vi "AlGaInPAs_prep_run_cont_v09.vi"(2 "Debug Mode":bool, 3 "Elapsed Time(s)":dbl, 4 "State":enum16{"Edit", "Start", "Run", "End", "Idle"}(ring), 5 "Argument List In":string[](array[string])) -> (0 "Status Out":string, 1 "Argument List Out":string[](array[string]))   [LabVIEW 2011]
panel:
  out "prep_done":bool
  out "run started":bool
  out "first":bool=TRUE
  out "total time":dbl
  out "is OK?":bool
  out "AsH3?":bool
  out "PH3?":bool
  out "In?":bool
  out "Ga?":bool
  out "Al?":bool
  in  "Prep As":bool caption="Pre-run"
  in  "Prep P":bool caption="Pre-run"
  in  "Prep In":bool caption="Pre-run"
  in  "Prep Ga":bool caption="Pre-run"
  in  "prep_time":dbl caption="pre-run time (s)"
  in  "Prep Al":bool caption="Pre-run"
  in  "Run As":bool caption="Run"
  in  "AsH3 Flow":dbl caption="AsH3 Flow (0-10 sccm)" format="%.2f"
  in  "P Flow":dbl caption="P Flow (0-100 sccm)" format="%.2f"
  in  "Run P":bool caption="Run"
  in  "In Flow":dbl caption="In Flow (0-100 sscm)" format="%.2f"
  in  "Run In":bool caption="Run"
  in  "Run Ga":bool caption="Run"
  in  "Ga Flow":dbl caption="Ga Flow (0-10 sscm)" format="%.2f"
  in  "Run Al":bool caption="Run"
  in  "Al Flow":dbl caption="Al Flow (0-100 sscm)" format="%.2f"
  in  "Cancel":bool
  in  "OK":bool
  out "tTotal(s) 2":dbl
  # "Add pre-run time to run time in editor."
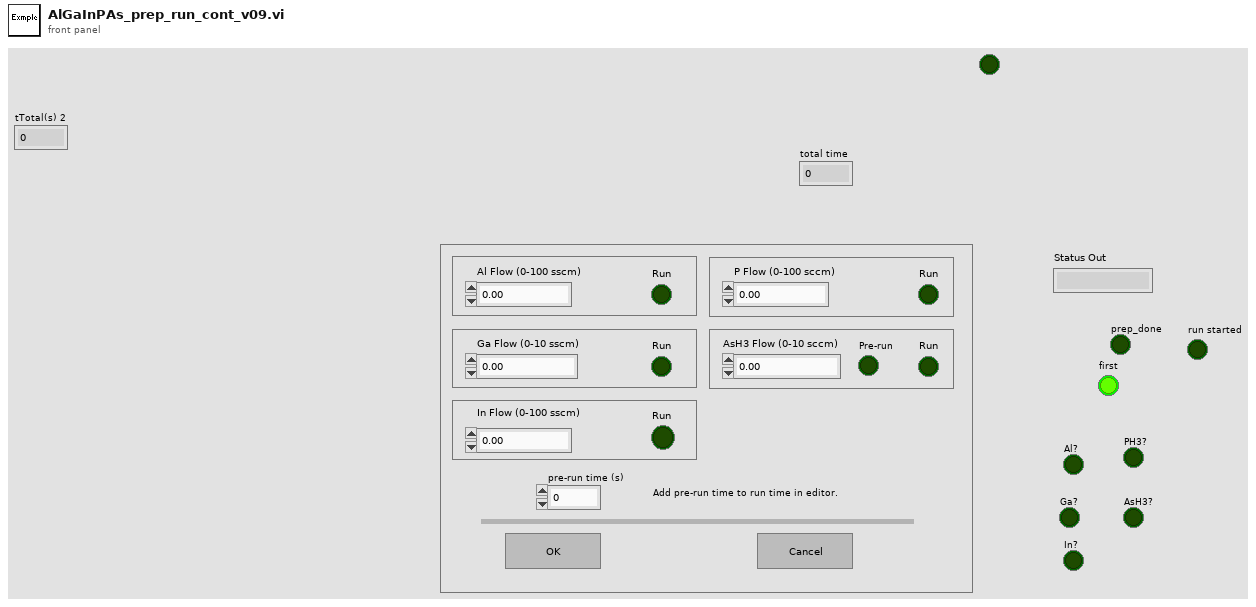
[diagram p1: front panel]
types:
  T1 = enum16{"Discrete", "Continuous", "Instantaneous", "Finite"}
  T2 = enum32{"Invalid", "Default", "Floating", "Floating/Auto-Hide", "Modal"}
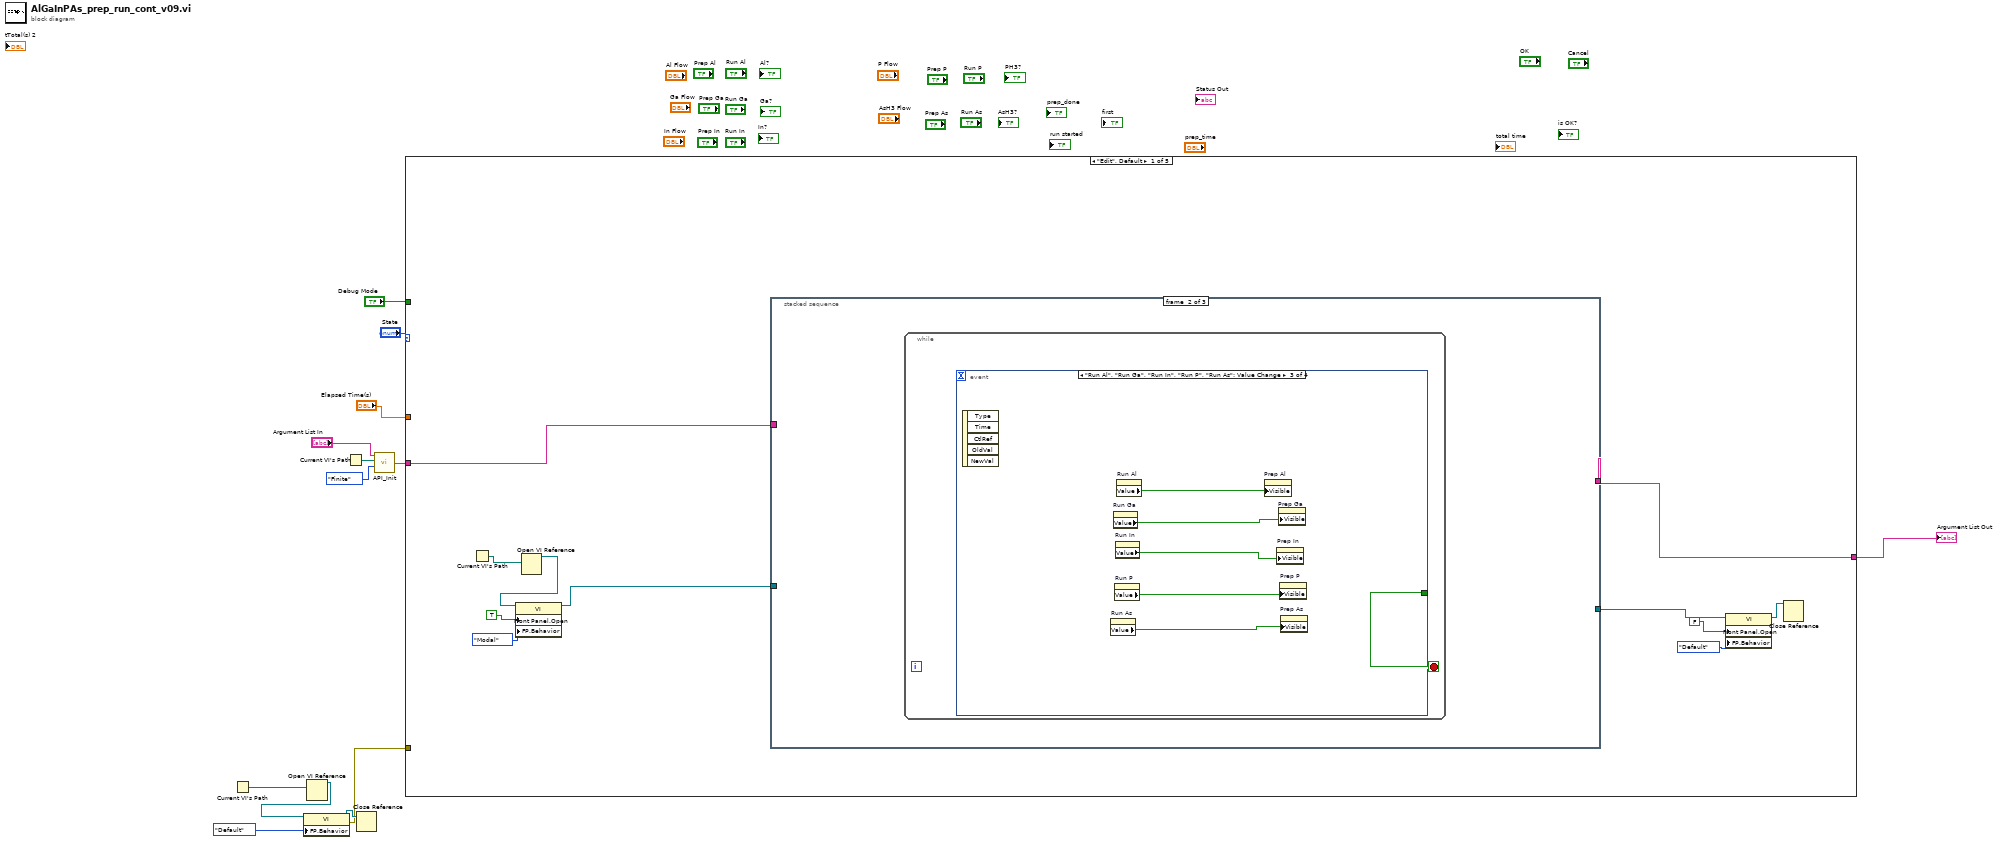
[diagram p0: block diagram]
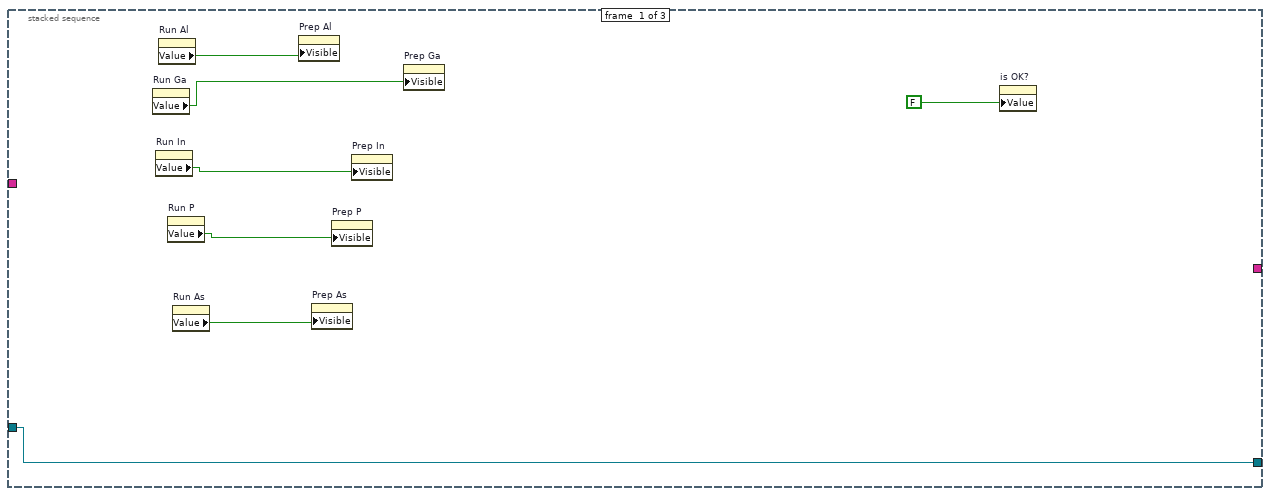
[diagram p2: hidden frame]
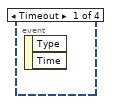
[diagram p3: hidden frame]
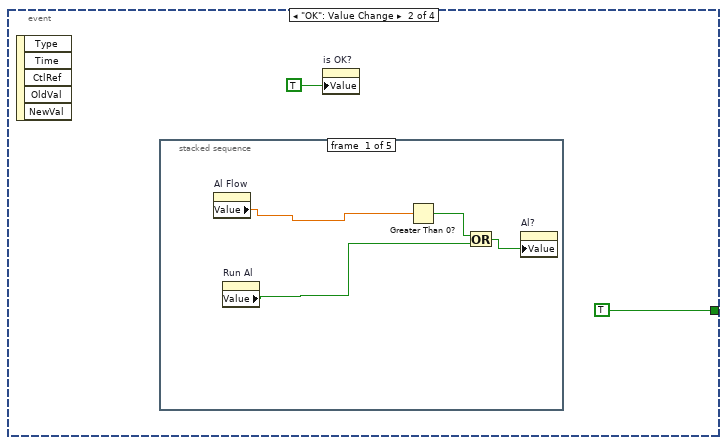
[diagram p4: hidden frame]
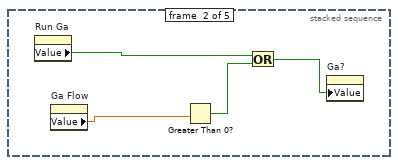
[diagram p5: hidden frame]
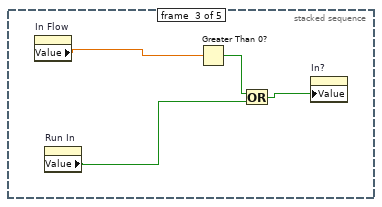
[diagram p6: hidden frame]
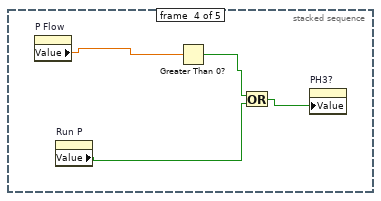
[diagram p7: hidden frame]
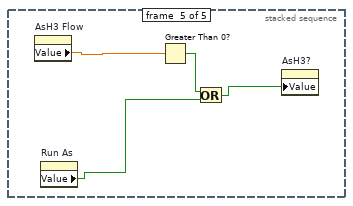
[diagram p8: hidden frame]
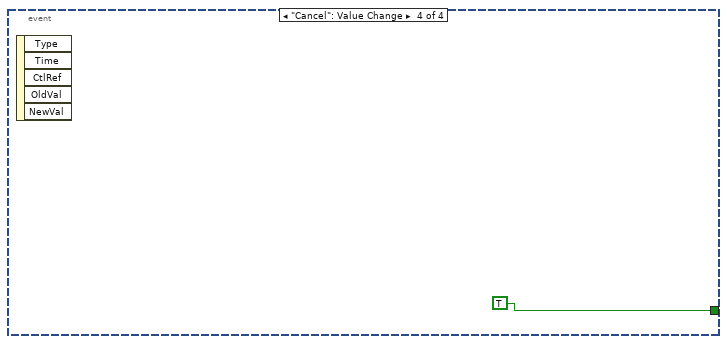
[diagram p9: hidden frame]
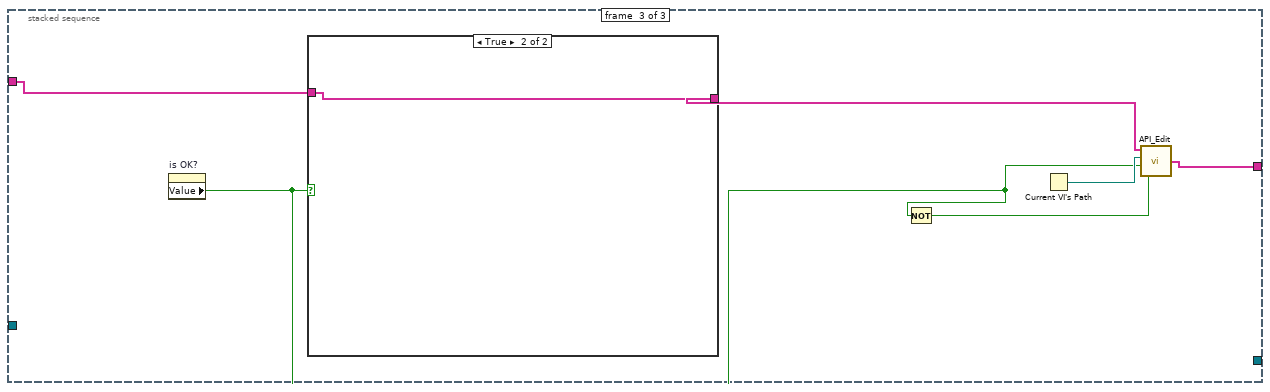
[diagram p10: hidden frame]
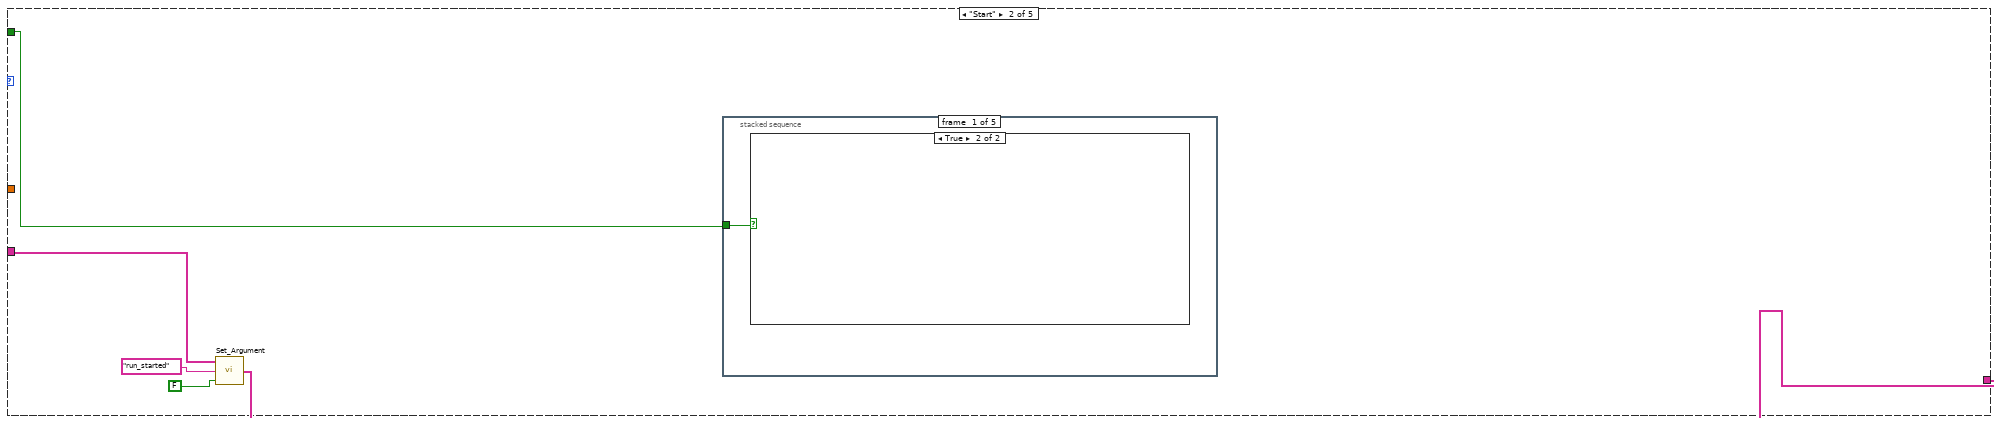
[diagram p12: hidden frame]
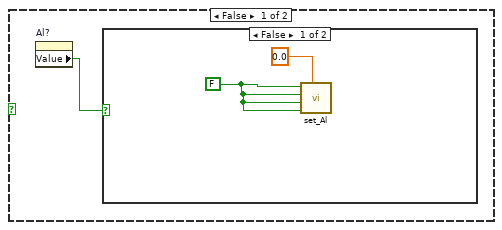
[diagram p13: hidden frame]
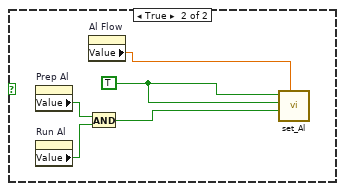
[diagram p14: hidden frame]
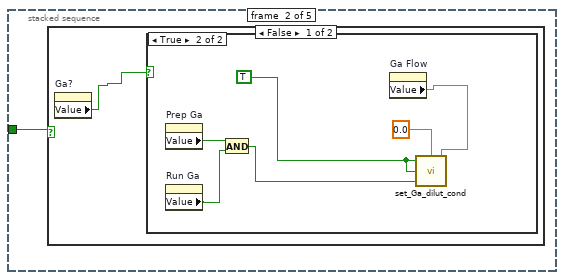
[diagram p15: hidden frame]
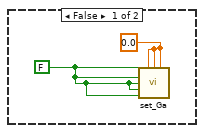
[diagram p16: hidden frame]
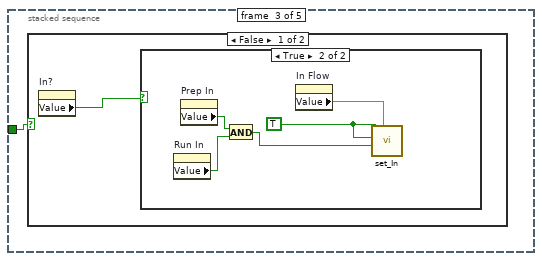
[diagram p18: hidden frame]
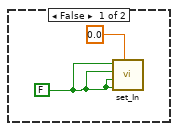
[diagram p19: hidden frame]
diagram:
  n1 = Current VI's Path() -> (path=w9:path)
  n2 = Open VI Reference(vi path=w9) -> (vi reference=w8:refnum<vi>)  [unwired: 1 in, 5 out]
  n3 = property class="VI"(reference=w8, "FP.Behavior"=T2."Default" ("Front Panel Window:Behavior")) -> (reference out=w6:refnum<vi>, error out=w5:errorcluster)  [unwired: 1 in]
  n4 = Current VI's Path() -> (path=w4:path)
  n5 = Close Reference(reference=w6) -> ()  [unwired: 1 in, 1 out]
  n6 = call "API_Init.vi"("API Mode"=T1."Finite", "VI Path"=w4, "Argument List In"="Argument List In") -> ("Argument List Out"=w1:string[])  [unwired: 1 in]
  n7 = case shown="\"Edit\", Default" "State" {
    tunnel: "Debug Mode" -> [_ w69 w121 _ _]
    tunnel: "Elapsed Time(s)" -> [_ _ w123 _ _]
    tunnel: w1 -> [w15 w71 w120 w236 w237]
    tunnel: [w14 w70 w122 w236 w237] -> w10
    tunnel: w5 -> [_ _ _ _ _]
    frame "Edit", Default {
      n8 = Current VI's Path() -> (path=w20:path)
      n9 = Open VI Reference(vi path=w20) -> (vi reference=w19:refnum<vi>)  [unwired: 1 in, 5 out]
      n10 = property class="VI"(reference=w19, "Front Panel.Open"=TRUE ("Front Panel Window:Open"), "FP.Behavior"=T2."Modal" ("Front Panel Window:Behavior")) -> (reference out=w18:refnum<vi>)  [unwired: 1 in, 1 out]
      n11 = stacked-sequence {
        tunnel: w15 -> [_ _ w64]
        tunnel: w18 -> [w31 _ _]
        tunnel: [w31 _ _] -> w22
        tunnel: [_ _ w62] -> w14
        frame #0 {
          n12 = property on="Run Ga" class="Bool (strict)"() -> ("Value"=w28:bool)  [unwired: 2 in, 2 out]
          n13 = property on="Run In" class="Bool (strict)"() -> ("Value"=w27:bool)  [unwired: 2 in, 2 out]
          n14 = property on="Run Al" class="Bool (strict)"() -> ("Value"=w29:bool)  [unwired: 2 in, 2 out]
          n15 = property on="Run P" class="Bool (strict)"() -> ("Value"=w26:bool)  [unwired: 2 in, 2 out]
          n16 = property on="Run As" class="Bool (strict)"() -> ("Value"=w25:bool)  [unwired: 2 in, 2 out]
          n17 = property on="Prep Al" class="Bool (strict)"("Visible"=w29) -> ()  [unwired: 2 in, 2 out]
          n18 = property on="Prep As" class="Bool (strict)"("Visible"=w25) -> ()  [unwired: 2 in, 2 out]
          n19 = property on="Prep P" class="Bool (strict)"("Visible"=w26) -> ()  [unwired: 2 in, 2 out]
          n20 = property on="Prep In" class="Bool (strict)"("Visible"=w27) -> ()  [unwired: 2 in, 2 out]
          n21 = property on="Prep Ga" class="Bool (strict)"("Visible"=w28) -> ()  [unwired: 2 in, 2 out]
          n22 = property on="is OK?" class="Bool (strict)"("Value"=FALSE ("is OK?")) -> ()  [unwired: 2 in, 2 out]
        }
        frame #1 {
          n23 = while {
            stop <- w32 stop-if-true
            n24 = event shown="[2] \"Run Al\", \"Run Ga\", \"Run In\", \"Run P\", \"Run As\": Value Change" {
              selector: _ -> [_ _ _ _]
              dyn-events: _ -> [_ _ _ _]
              timeout: _ -> [_ _ _ _]
              tunnel: [_ TRUE _ TRUE] -> w32
              event Timeout {
                n25 = event-data() -> ()  [unwired: 1 in, 2 out]
              }
              event "OK": Value Change {
                n26 = event-data() -> ()  [unwired: 1 in, 5 out]
                n27 = stacked-sequence {
                  frame #0 {
                    n28 = property on="Al Flow" class="DigNum (strict)"() -> ("Value"=w37:dbl)  [unwired: 2 in, 2 out]
                    n29 = property on="Run Al" class="Bool (strict)"() -> ("Value"=w36:bool)  [unwired: 2 in, 2 out]
                    n30 = Greater Than 0?(x=w37) -> (x > 0?=w38:bool)
                    n31 = Or(x=w38, y=w36) -> (x .or. y?=w35:bool)
                    n32 = property on="Al?" class="Bool (strict)"("Value"=w35) -> ()  [unwired: 2 in, 2 out]
                  }
                  frame #1 {
                    n33 = property on="Run Ga" class="Bool (strict)"() -> ("Value"=w40:bool)  [unwired: 2 in, 2 out]
                    n34 = property on="Ga Flow" class="DigNum (strict)"() -> ("Value"=w41:dbl)  [unwired: 2 in, 2 out]
                    n35 = Greater Than 0?(x=w41) -> (x > 0?=w42:bool)
                    n36 = Or(x=w40, y=w42) -> (x .or. y?=w39:bool)
                    n37 = property on="Ga?" class="Bool (strict)"("Value"=w39) -> ()  [unwired: 2 in, 2 out]
                  }
                  frame #2 {
                    n38 = property on="In Flow" class="DigNum (strict)"() -> ("Value"=w44:dbl)  [unwired: 2 in, 2 out]
                    n39 = property on="Run In" class="Bool (strict)"() -> ("Value"=w45:bool)  [unwired: 2 in, 2 out]
                    n40 = Greater Than 0?(x=w44) -> (x > 0?=w46:bool)
                    n41 = Or(x=w46, y=w45) -> (x .or. y?=w43:bool)
                    n42 = property on="In?" class="Bool (strict)"("Value"=w43) -> ()  [unwired: 2 in, 2 out]
                  }
                  frame #3 {
                    n43 = property on="P Flow" class="DigNum (strict)"() -> ("Value"=w49:dbl)  [unwired: 2 in, 2 out]
                    n44 = property on="Run P" class="Bool (strict)"() -> ("Value"=w48:bool)  [unwired: 2 in, 2 out]
                    n45 = Greater Than 0?(x=w49) -> (x > 0?=w50:bool)
                    n46 = Or(x=w50, y=w48) -> (x .or. y?=w47:bool)
                    n47 = property on="PH3?" class="Bool (strict)"("Value"=w47) -> ()  [unwired: 2 in, 2 out]
                  }
                  frame #4 {
                    n48 = property on="AsH3 Flow" class="DigNum (strict)"() -> ("Value"=w53:dbl)  [unwired: 2 in, 2 out]
                    n49 = property on="Run As" class="Bool (strict)"() -> ("Value"=w52:bool)  [unwired: 2 in, 2 out]
                    n50 = Greater Than 0?(x=w53) -> (x > 0?=w54:bool)
                    n51 = Or(x=w54, y=w52) -> (x .or. y?=w51:bool)
                    n52 = property on="AsH3?" class="Bool (strict)"("Value"=w51) -> ()  [unwired: 2 in, 2 out]
                  }
                }
                n53 = property on="is OK?" class="Bool (strict)"("Value"=TRUE ("is OK?")) -> ()  [unwired: 2 in, 2 out]
              }
              event "Run Al", "Run Ga", "Run In", "Run P", "Run As": Value Change {
                n54 = event-data() -> ()  [unwired: 1 in, 5 out]
                n55 = property on="Run As" class="Bool (strict)"() -> ("Value"=w59:bool)  [unwired: 2 in, 2 out]
                n56 = property on="Run Ga" class="Bool (strict)"() -> ("Value"=w56:bool)  [unwired: 2 in, 2 out]
                n57 = property on="Run P" class="Bool (strict)"() -> ("Value"=w58:bool)  [unwired: 2 in, 2 out]
                n58 = property on="Run In" class="Bool (strict)"() -> ("Value"=w57:bool)  [unwired: 2 in, 2 out]
                n59 = property on="Run Al" class="Bool (strict)"() -> ("Value"=w55:bool)  [unwired: 2 in, 2 out]
                n60 = property on="Prep Al" class="Bool (strict)"("Visible"=w55) -> ()  [unwired: 2 in, 2 out]
                n61 = property on="Prep In" class="Bool (strict)"("Visible"=w57) -> ()  [unwired: 2 in, 2 out]
                n62 = property on="Prep Ga" class="Bool (strict)"("Visible"=w56) -> ()  [unwired: 2 in, 2 out]
                n63 = property on="Prep P" class="Bool (strict)"("Visible"=w58) -> ()  [unwired: 2 in, 2 out]
                n64 = property on="Prep As" class="Bool (strict)"("Visible"=w59) -> ()  [unwired: 2 in, 2 out]
              }
              event "Cancel": Value Change {
                n65 = event-data() -> ()  [unwired: 1 in, 5 out]
              }
            }
          }
        }
        frame #2 {
          n66 = property on="is OK?" class="Bool (strict)"() -> ("Value"=w61:bool)  [unwired: 2 in, 2 out]
          n67 = case shown="True" w61 {
            tunnel: w64 -> [w67 w68]
            tunnel: [w67 w68] -> w63
            frame False {
            }
            frame True {
            }
          }
          n68 = Not(x=w61) -> (.not. x?=w66:bool)
          n69 = Current VI's Path() -> (path=w65:path)
          n70 = call "API_Edit.vi"("Cancel"=w66, "OK"=w61, "VI Path"=w65, "Argument List In"=w63) -> ("Argument List Out"=w62:string[])
        }
      }
      n71 = property class="VI"(reference=w22, "Front Panel.Open"=FALSE ("Front Panel Window:Open"), "FP.Behavior"=T2."Default" ("Front Panel Window:Behavior")) -> (reference out=w23:refnum<vi>)  [unwired: 1 in, 1 out]
      n72 = Close Reference(reference=w23) -> ()  [unwired: 1 in, 1 out]
    }
    frame "Start" {
      n73 = call "Set_Argument.vi"("Enable"=FALSE, "Argument"="run_started", "Argument List In"=w71) -> ("Argument List Out"=w70:string[])
      n74 = stacked-sequence {
        tunnel: w69 -> [w74 w83 w93 w102 w111]
        frame #0 {
          n75 = case shown="True" w74 {
            frame False {
              n76 = property on="Al?" class="Bool (strict)"() -> ("Value"=w75:bool)  [unwired: 2 in, 2 out]
              n77 = case shown="False" w75 {
                frame False {
                  w76 = FALSE ("Al Active")
                  n78 = call "set_Al.vi"("Aluminum Flow"=0.0, "Al Remote"=w76, "Al Run"=w76, "Al Bubbler"=w76, "Al Active"=w76) -> ()  [unwired: 5 out]
                }
                frame True {
                  w82 = TRUE ("Al Active")
                  n79 = property on="Prep Al" class="Bool (strict)"() -> ("Value"=w80:bool)  [unwired: 2 in, 2 out]
                  n80 = property on="Run Al" class="Bool (strict)"() -> ("Value"=w79:bool)  [unwired: 2 in, 2 out]
                  n81 = property on="Al Flow" class="DigNum (strict)"() -> ("Value"=w81:dbl)  [unwired: 2 in, 2 out]
                  n82 = And(x=w80, y=w79) -> (x .and. y?=w78:bool)
                  n83 = call "set_Al.vi"("Aluminum Flow"=w81, "Al Run"=w78, "Al Bubbler"=w82, "Al Active"=w82) -> ()  [unwired: 1 in, 5 out]
                }
              }
            }
            frame True {
            }
          }
        }
        frame #1 {
          n84 = case shown="False" w83 {
            frame False {
              n85 = property on="Ga?" class="Bool (strict)"() -> ("Value"=w84:bool)  [unwired: 2 in, 2 out]
              n86 = case shown="True" w84 {
                frame False {
                  w86 = FALSE ("Ga Active")
                  w85 = 0.0 ("Ga Flow 1")
                  n87 = call "set_Ga.vi"("Ga Active"=w86, "Ga Flow 3"=w85, "Ga Flow 2"=w85, "Ga Flow 1"=w85, "Ga Bubbler"=w86, "Ga H2 Dilute"=w86, "Ga Run"=w86, "Ga Remote"=w86) -> ()  [unwired: 8 out]
                }
                frame True {
                  w92 = TRUE ("Ga Active")
                  n88 = property on="Prep Ga" class="Bool (strict)"() -> ("Value"=w89:bool)  [unwired: 2 in, 2 out]
                  n89 = property on="Run Ga" class="Bool (strict)"() -> ("Value"=w88:bool)  [unwired: 2 in, 2 out]
                  n90 = And(x=w89, y=w88) -> (x .and. y?=w87:bool)
                  n91 = property on="Ga Flow" class="DigNum (strict)"() -> ("Value"=w90:dbl)  [unwired: 2 in, 2 out]
                  n92 = call "set_Ga_dilut_cond.vi"("Ga flow (0-10 sccm)"=w90, "fDilution"=0.0, "Run"=w87, "Bubbler In"=w92, "Active"=w92) -> ()
                }
              }
            }
            frame True {
            }
          }
        }
        frame #2 {
          n93 = case shown="False" w93 {
            frame False {
              n94 = property on="In?" class="Bool (strict)"() -> ("Value"=w94:bool)  [unwired: 2 in, 2 out]
              n95 = case shown="True" w94 {
                frame False {
                  w96 = FALSE ("In Remote")
                  n96 = call "set_In.vi"("Indium Flow"=0.0, "In Remote"=w96, "In Run"=w96, "In Bubbler"=w96, "In Active"=w96) -> ()  [unwired: 5 out]
                }
                frame True {
                  w101 = TRUE ("In Run")
                  n97 = property on="Run In" class="Bool (strict)"() -> ("Value"=w98:bool)  [unwired: 2 in, 2 out]
                  n98 = property on="Prep In" class="Bool (strict)"() -> ("Value"=w99:bool)  [unwired: 2 in, 2 out]
                  n99 = And(x=w99, y=w98) -> (x .and. y?=w97:bool)
                  n100 = property on="In Flow" class="DigNum (strict)"() -> ("Value"=w100:dbl)  [unwired: 2 in, 2 out]
                  n101 = call "set_In.vi"("Indium Flow"=w100, "In Run"=w97, "In Bubbler"=w101, "In Active"=w101) -> ()  [unwired: 1 in, 5 out]
                }
              }
            }
            frame True {
            }
          }
        }
        frame #3 {
          n102 = case shown="False" w102 {
            frame False {
              n103 = property on="PH3?" class="Bool (strict)"() -> ("Value"=w103:bool)  [unwired: 2 in, 2 out]
              n104 = case shown="True" w103 {
                frame False {
                  w104 = FALSE ("P_Gas Active")
                  n105 = call "set_P_gas.vi"("P_Gas Active"=w104, "P_Gas Flow"=0.0, "P_Gas In"=w104, "P_Gas H2 In"=w104, "P_Gas Run"=w104, "P_Gas Remote"=w104) -> ()  [unwired: 10 out]
                }
                frame True {
                  w110 = TRUE ("P_Gas Active")
                  n106 = property on="P Flow" class="DigNum (strict)"() -> ("Value"=w109:dbl)  [unwired: 2 in, 2 out]
                  n107 = property on="Prep P" class="Bool (strict)"() -> ("Value"=w108:bool)  [unwired: 2 in, 2 out]
                  n108 = property on="Run P" class="Bool (strict)"() -> ("Value"=w107:bool)  [unwired: 2 in, 2 out]
                  n109 = And(x=w108, y=w107) -> (x .and. y?=w106:bool)
                  n110 = call "set_P_gas.vi"("P_Gas Active"=w110, "P_Gas Flow"=w109, "P_Gas In"=w110, "P_Gas Run"=w106) -> ()  [unwired: 2 in, 10 out]
                }
              }
            }
            frame True {
            }
          }
        }
        frame #4 {
          n111 = case shown="False" w111 {
            frame False {
              n112 = property on="AsH3?" class="Bool (strict)"() -> ("Value"=w112:bool)  [unwired: 2 in, 2 out]
              n113 = case shown="True" w112 {
                frame False {
                  w113 = FALSE ("As_Gas Active")
                  n114 = call "set_As_gas.vi"("As_Gas Active"=w113, "As_Gas Flow"=0.0, "As_Gas In"=w113, "As_Gas H2"=w113, "As_Gas Run"=w113, "As_Gas Remote"=w113) -> ()  [unwired: 10 in]
                }
                frame True {
                  w119 = TRUE ("As_Gas Active")
                  n115 = property on="Prep As" class="Bool (strict)"() -> ("Value"=w116:bool)  [unwired: 2 in, 2 out]
                  n116 = property on="Run As" class="Bool (strict)"() -> ("Value"=w117:bool)  [unwired: 2 in, 2 out]
                  n117 = property on="AsH3 Flow" class="DigNum (strict)"() -> ("Value"=w118:dbl)  [unwired: 2 in, 2 out]
                  n118 = And(x=w116, y=w117) -> (x .and. y?=w115:bool)
                  n119 = call "set_As_gas.vi"("As_Gas Active"=w119, "As_Gas Flow"=w118, "As_Gas In"=w119, "As_Gas Run"=w115) -> ()  [unwired: 12 in]
                }
              }
            }
            frame True {
            }
          }
        }
      }
    }
    frame "Run" {
      n120 = stacked-sequence {
        tunnel: w123 -> [_ w128 _ _]
        tunnel: w120 -> [w125 _ _ w182]
        tunnel: [_ _ _ w181] -> w122
        tunnel: w121 -> [_ _ _ w183]
        frame #0 {
          n121 = call "Get_Argument.vi"("Argument"="run_started", "Argument List"=w125) -> ("Enabled"=w124:bool)
          n122 = local write "run started"(w124) -> ()
        }
        frame #1 {
          n123 = property on="prep_time" class="DigNum (strict)"() -> ("Value"=w129:dbl)  [unwired: 2 in, 2 out]
          n124 = Greater Or Equal?(x=w128, y=w129) -> (x >= y?=w127:bool)
          n125 = local write "prep_done"(w127) -> ()
        }
        frame #2 {
          n126 = local read "run started"() -> (w131:bool)
          n127 = Not(x=w131) -> (.not. x?=w130:bool)
          n128 = stacked-sequence {
            tunnel: w130 -> [w133 w137 w146 w155 w164 w173]
            frame #0 {
              n129 = case shown="True" w133 {
                tunnel: ["run: " "pre-run: "] -> w132
                frame False {
                }
                frame True {
                }
              }
              n130 = property on="Status Out" class="Str"("Value"=w132) -> ()  [unwired: 2 in, 2 out]
            }
            frame #1 {
              n131 = property on="Status Out" class="Str"() -> ("Value"=w143:string)  [unwired: 2 in, 2 out]
              n132 = property on="Al?" class="Bool (strict)"() -> ("Value"=w144:bool)  [unwired: 2 in, 2 out]
              n133 = property on="Run Al" class="Bool (strict)"() -> ("Value"=w136:bool)  [unwired: 2 in, 2 out]
              n134 = property on="Prep Al" class="Bool (strict)"() -> ("Value"=w138:bool)  [unwired: 2 in, 2 out]
              n135 = call "flow_strings.vi"("string in"=w143, "is first in?"=TRUE, "use source?"=w144, "name"="Al", "run source?"=w136, "prep source?"=w138, "is prep?"=w137) -> ("string out"=w142:string, "is first out?"=w141:bool)
              n136 = property on="Status Out" class="Str"("Value"=w142) -> ()  [unwired: 2 in, 2 out]
              n137 = property on="first" class="Bool (strict)"("Value"=w141) -> ()  [unwired: 2 in, 2 out]
            }
            frame #2 {
              n138 = property on="first" class="Bool (strict)"() -> ("Value"=w149:bool)  [unwired: 2 in, 2 out]
              n139 = property on="Status Out" class="Str"() -> ("Value"=w152:string)  [unwired: 2 in, 2 out]
              n140 = property on="Ga?" class="Bool (strict)"() -> ("Value"=w150:bool)  [unwired: 2 in, 2 out]
              n141 = property on="Run Ga" class="Bool (strict)"() -> ("Value"=w145:bool)  [unwired: 2 in, 2 out]
              n142 = property on="Prep Ga" class="Bool (strict)"() -> ("Value"=w147:bool)  [unwired: 2 in, 2 out]
              n143 = call "flow_strings.vi"("string in"=w152, "is first in?"=w149, "use source?"=w150, "name"="Ga", "run source?"=w145, "prep source?"=w147, "is prep?"=w146) -> ("string out"=w153:string, "is first out?"=w148:bool)
              n144 = property on="Status Out" class="Str"("Value"=w153) -> ()  [unwired: 2 in, 2 out]
              n145 = property on="first" class="Bool (strict)"("Value"=w148) -> ()  [unwired: 2 in, 2 out]
            }
            frame #3 {
              n146 = property on="first" class="Bool (strict)"() -> ("Value"=w159:bool)  [unwired: 2 in, 2 out]
              n147 = property on="Status Out" class="Str"() -> ("Value"=w161:string)  [unwired: 2 in, 2 out]
              n148 = property on="In?" class="Bool (strict)"() -> ("Value"=w162:bool)  [unwired: 2 in, 2 out]
              n149 = property on="Run In" class="Bool (strict)"() -> ("Value"=w154:bool)  [unwired: 2 in, 2 out]
              n150 = property on="Prep In" class="Bool (strict)"() -> ("Value"=w156:bool)  [unwired: 2 in, 2 out]
              n151 = call "flow_strings.vi"("string in"=w161, "is first in?"=w159, "use source?"=w162, "name"="In", "run source?"=w154, "prep source?"=w156, "is prep?"=w155) -> ("string out"=w158:string, "is first out?"=w157:bool)
              n152 = property on="Status Out" class="Str"("Value"=w158) -> ()  [unwired: 2 in, 2 out]
              n153 = property on="first" class="Bool (strict)"("Value"=w157) -> ()  [unwired: 2 in, 2 out]
            }
            frame #4 {
              n154 = property on="first" class="Bool (strict)"() -> ("Value"=w167:bool)  [unwired: 2 in, 2 out]
              n155 = property on="Status Out" class="Str"() -> ("Value"=w169:string)  [unwired: 2 in, 2 out]
              n156 = property on="PH3?" class="Bool (strict)"() -> ("Value"=w170:bool)  [unwired: 2 in, 2 out]
              n157 = property on="Run P" class="Bool (strict)"() -> ("Value"=w163:bool)  [unwired: 2 in, 2 out]
              n158 = property on="Prep P" class="Bool (strict)"() -> ("Value"=w165:bool)  [unwired: 2 in, 2 out]
              n159 = call "flow_strings.vi"("string in"=w169, "is first in?"=w167, "use source?"=w170, "name"="P", "run source?"=w163, "prep source?"=w165, "is prep?"=w164) -> ("string out"=w168:string, "is first out?"=w166:bool)
              n160 = property on="Status Out" class="Str"("Value"=w168) -> ()  [unwired: 2 in, 2 out]
              n161 = property on="first" class="Bool (strict)"("Value"=w166) -> ()  [unwired: 2 in, 2 out]
            }
            frame #5 {
              n162 = property on="first" class="Bool (strict)"() -> ("Value"=w176:bool)  [unwired: 2 in, 2 out]
              n163 = property on="Status Out" class="Str"() -> ("Value"=w178:string)  [unwired: 2 in, 2 out]
              n164 = property on="AsH3?" class="Bool (strict)"() -> ("Value"=w179:bool)  [unwired: 2 in, 2 out]
              n165 = property on="Run As" class="Bool (strict)"() -> ("Value"=w172:bool)  [unwired: 2 in, 2 out]
              n166 = property on="Prep As" class="Bool (strict)"() -> ("Value"=w174:bool)  [unwired: 2 in, 2 out]
              n167 = call "flow_strings.vi"("string in"=w178, "is first in?"=w176, "use source?"=w179, "name"="As", "run source?"=w172, "prep source?"=w174, "is prep?"=w173) -> ("string out"=w175:string, "is first out?"=w177:bool)
              n168 = property on="Status Out" class="Str"("Value"=w175) -> ()  [unwired: 2 in, 2 out]
              n169 = property on="first" class="Bool (strict)"("Value"=w177) -> ()  [unwired: 2 in, 2 out]
            }
          }
        }
        frame #3 {
          n170 = local read "run started"() -> (w186:bool)
          n171 = local read "prep_done"() -> (w184:bool)
          n172 = Not(x=w186) -> (.not. x?=w187:bool)
          n173 = And(x=w184, y=w187) -> (x .and. y?=w185:bool)
          n174 = stacked-sequence {
            tunnel: w185 -> [w191]
            tunnel: w183 -> [w190]
            tunnel: w182 -> [w189]
            tunnel: [w188] -> w181
            frame #0 {
              n175 = case shown="True" w191 {
                tunnel: w190 -> [_ w195]
                tunnel: w189 -> [w192 w194]
                tunnel: [w192 w193] -> w188
                frame False {
                }
                frame True {
                  n176 = stacked-sequence {
                    tunnel: w195 -> [w196 w203 w211 w218 w225 _]
                    tunnel: w194 -> [_ _ _ _ _ w233]
                    tunnel: [_ _ _ _ _ w232] -> w193
                    frame #0 {
                      n177 = case shown="False" w196 {
                        frame False {
                          n178 = property on="Al?" class="Bool (strict)"() -> ("Value"=w197:bool)  [unwired: 2 in, 2 out]
                          n179 = case shown="True" w197 {
                            frame False {
                              w198 = FALSE ("Al Active")
                              n180 = call "set_Al.vi"("Aluminum Flow"=0.0, "Al Remote"=w198, "Al Run"=w198, "Al Bubbler"=w198, "Al Active"=w198) -> ()  [unwired: 5 out]
                            }
                            frame True {
                              w202 = TRUE ("Al Active")
                              n181 = property on="Al Flow" class="DigNum (strict)"() -> ("Value"=w201:dbl)  [unwired: 2 in, 2 out]
                              n182 = property on="Run Al" class="Bool (strict)"() -> ("Value"=w200:bool)  [unwired: 2 in, 2 out]
                              n183 = call "set_Al.vi"("Aluminum Flow"=w201, "Al Run"=w200, "Al Bubbler"=w202, "Al Active"=w202) -> ()  [unwired: 1 in, 5 out]
                            }
                          }
                        }
                        frame True {
                        }
                      }
                    }
                    frame #1 {
                      n184 = case shown="False" w203 {
                        frame False {
                          n185 = property on="Ga?" class="Bool (strict)"() -> ("Value"=w204:bool)  [unwired: 2 in, 2 out]
                          n186 = case shown="False" w204 {
                            frame False {
                              w206 = FALSE ("Ga Active")
                              w205 = 0.0 ("Ga Flow 1")
                              n187 = call "set_Ga.vi"("Ga Active"=w206, "Ga Flow 3"=w205, "Ga Flow 2"=w205, "Ga Flow 1"=w205, "Ga Bubbler"=w206, "Ga H2 Dilute"=w206, "Ga Run"=w206, "Ga Remote"=w206) -> ()  [unwired: 8 out]
                            }
                            frame True {
                              w210 = TRUE ("Ga Active")
                              n188 = property on="Ga Flow" class="DigNum (strict)"() -> ("Value"=w207:dbl)  [unwired: 2 in, 2 out]
                              n189 = property on="Run Ga" class="Bool (strict)"() -> ("Value"=w208:bool)  [unwired: 2 in, 2 out]
                              n190 = call "set_Ga_dilut_cond.vi"("Ga flow (0-10 sccm)"=w207, "fDilution"=0.0, "Run"=w208, "Bubbler In"=w210, "Active"=w210) -> ()
                            }
                          }
                        }
                        frame True {
                        }
                      }
                    }
                    frame #2 {
                      n191 = case shown="False" w211 {
                        frame False {
                          n192 = property on="In?" class="Bool (strict)"() -> ("Value"=w212:bool)  [unwired: 2 in, 2 out]
                          n193 = case shown="True" w212 {
                            frame False {
                              w214 = FALSE ("In Remote")
                              n194 = call "set_In.vi"("Indium Flow"=0.0, "In Remote"=w214, "In Run"=w214, "In Bubbler"=w214, "In Active"=w214) -> ()  [unwired: 5 out]
                            }
                            frame True {
                              w217 = TRUE ("In Run")
                              n195 = property on="Run In" class="Bool (strict)"() -> ("Value"=w215:bool)  [unwired: 2 in, 2 out]
                              n196 = property on="In Flow" class="DigNum (strict)"() -> ("Value"=w216:dbl)  [unwired: 2 in, 2 out]
                              n197 = call "set_In.vi"("Indium Flow"=w216, "In Run"=w215, "In Bubbler"=w217, "In Active"=w217) -> ()  [unwired: 1 in, 5 out]
                            }
                          }
                        }
                        frame True {
                        }
                      }
                    }
                    frame #3 {
                      n198 = case shown="False" w218 {
                        frame False {
                          n199 = property on="PH3?" class="Bool (strict)"() -> ("Value"=w219:bool)  [unwired: 2 in, 2 out]
                          n200 = case shown="False" w219 {
                            frame False {
                              w220 = FALSE ("P_Gas Active")
                              n201 = call "set_P_gas.vi"("P_Gas Active"=w220, "P_Gas Flow"=0.0, "P_Gas In"=w220, "P_Gas H2 In"=w220, "P_Gas Run"=w220, "P_Gas Remote"=w220) -> ()  [unwired: 10 out]
                            }
                            frame True {
                              w224 = TRUE ("P_Gas Active")
                              n202 = property on="P Flow" class="DigNum (strict)"() -> ("Value"=w223:dbl)  [unwired: 2 in, 2 out]
                              n203 = property on="Run P" class="Bool (strict)"() -> ("Value"=w222:bool)  [unwired: 2 in, 2 out]
                              n204 = call "set_P_gas.vi"("P_Gas Active"=w224, "P_Gas Flow"=w223, "P_Gas In"=w224, "P_Gas Run"=w222) -> ()  [unwired: 2 in, 10 out]
                            }
                          }
                        }
                        frame True {
                        }
                      }
                    }
                    frame #4 {
                      n205 = case shown="False" w225 {
                        frame False {
                          n206 = property on="AsH3?" class="Bool (strict)"() -> ("Value"=w226:bool)  [unwired: 2 in, 2 out]
                          n207 = case shown="True" w226 {
                            frame False {
                              w227 = FALSE ("As_Gas Active")
                              n208 = call "set_As_gas.vi"("As_Gas Active"=w227, "As_Gas Flow"=0.0, "As_Gas In"=w227, "As_Gas H2"=w227, "As_Gas Run"=w227, "As_Gas Remote"=w227) -> ()  [unwired: 10 in]
                            }
                            frame True {
                              w230 = TRUE ("As_Gas Active")
                              n209 = property on="Run As" class="Bool (strict)"() -> ("Value"=w229:bool)  [unwired: 2 in, 2 out]
                              n210 = property on="AsH3 Flow" class="DigNum (strict)"() -> ("Value"=w231:dbl)  [unwired: 2 in, 2 out]
                              n211 = call "set_As_gas.vi"("As_Gas Active"=w230, "As_Gas Flow"=w231, "As_Gas In"=w230, "As_Gas Run"=w229) -> ()  [unwired: 12 in]
                            }
                          }
                        }
                        frame True {
                        }
                      }
                    }
                    frame #5 {
                      n212 = call "Set_Argument.vi"("Enable"=TRUE, "Argument"="run_started", "Argument List In"=w233) -> ("Argument List Out"=w232:string[])
                    }
                  }
                }
              }
            }
          }
        }
      }
    }
    frame "End" {
    }
    frame "Idle" {
    }
  }
  "Argument List Out" <- w10
